vi "0036.vi"() -> ()   [LabVIEW 2014]
panel:
  out "測定中":bool
  in  "タブ制御器":enum32{"メイン画面", "設定"}(tab)
  out "XYグラフ":cluster{dbl[], dbl[]}[](graph)
  in  "再生ボタン":bool
  in  "停止ボタン":bool
  in  "全データ保存":bool
  out "経過時間":dbl format="%<%H:%M>t"
  out "数値出力":dbl format="%.1g"
  out "数値出力 2":dbl format="%.1g"
  out "数値出力 3":dbl format="%.1g"
  out "数値出力 4":dbl format="%.1g"
  out "数値出力 5":dbl format="%.1g"
  out "数値出力 6":dbl format="%.1g"
  in  "測定間隔（s）":dbl=5.0 min=5.0 step=5.0
  in  "終了時間（h）":dbl=9999.0 min=0.0 step=5.0
  out "稼働状態":bool
  out "停止合図":bool
  out "開始合図":bool
  in  "終了":bool
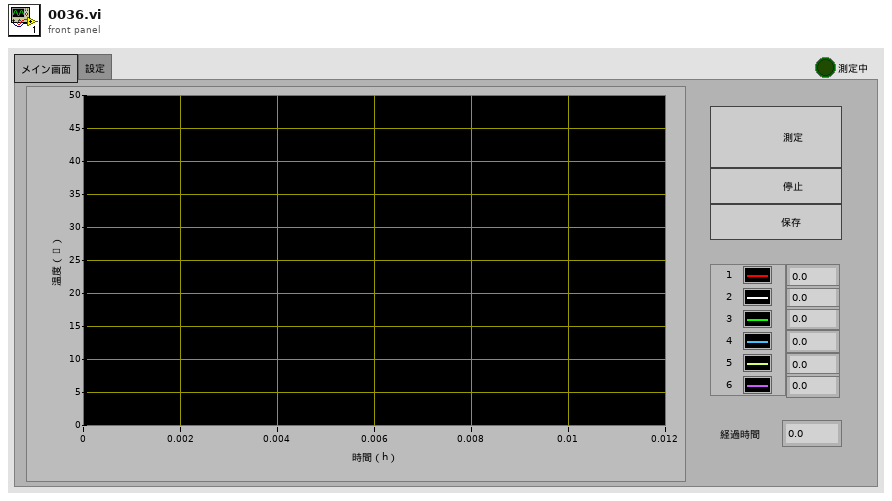
[diagram p1: front panel]
types:
  T1 = cluster{"bitRate":u32, "address":u8, "autoReadRespond":bool, "writeTimeout":u16, "readTimeout":u16, "sclLowTimeout":bool, "transferRetries":u16}
  T2 = typedef "CP2112_device.ctl" = i32
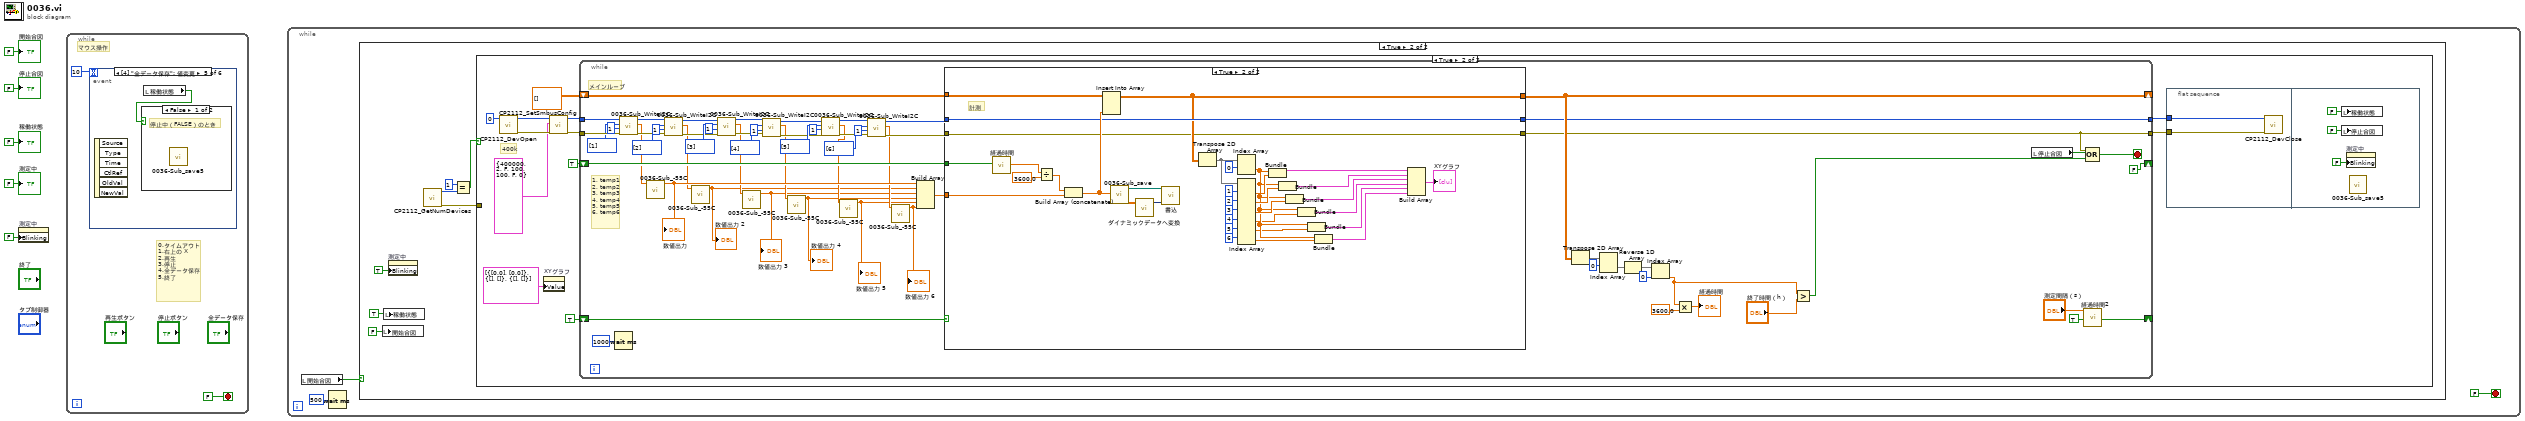
[diagram p0: block diagram]
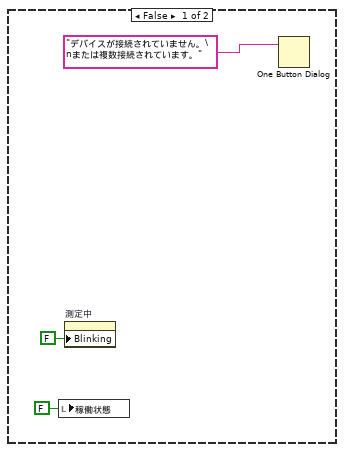
[diagram p3: hidden frame]
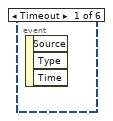
[diagram p5: hidden frame]
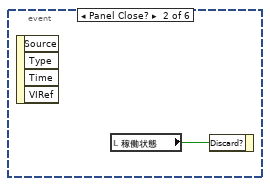
[diagram p6: hidden frame]
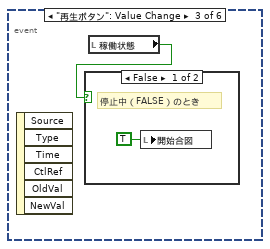
[diagram p7: hidden frame]
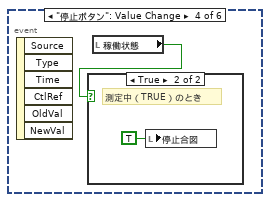
[diagram p9: hidden frame]
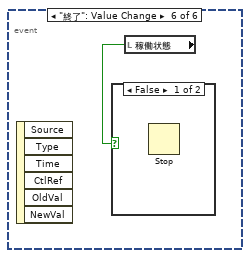
[diagram p12: hidden frame]
diagram:
  n1 = property on="測定中" class="Bool （指定）"("Blinking"=FALSE ("点滅")) -> ()  [unwired: 2 in, 2 out]
  n2 = while {
    stop <- FALSE stop-if-true
    # "マウス操作"
    # "0.タイムアウト\n1.右上の X\n2.再生\n3.停止\n4.全データ保存\n5.終了"
    n3 = event shown="[4] \"全データ保存\": 値変更" {
      selector: _ -> [_ _ _ _ _ _]
      dyn-events: _ -> [_ _ _ _ _ _]
      timeout: 10 -> [_ _ _ _ _ _]
      event Timeout {
        n4 = event-data() -> ()  [unwired: 1 in, 3 out]
      }
      event Panel Close? {
        n5 = event-data() -> ()  [unwired: 1 in, 4 out]
        n6 = local read "稼働状態"() -> (w8:bool)
        n7 = event-data("Discard?"=w8) -> ()  [unwired: 1 in, 1 out]
      }
      event "再生ボタン": Value Change {
        n8 = event-data() -> ()  [unwired: 1 in, 6 out]
        n9 = local read "稼働状態"() -> (w9:bool)
        n10 = case shown="FALSE" w9 {
          frame False {
            # "停止中（FALSE）のとき"
            n11 = local write "開始合図"(TRUE ("測定開始")) -> ()
          }
          frame True {
          }
        }
      }
      event "停止ボタン": Value Change {
        n12 = event-data() -> ()  [unwired: 1 in, 6 out]
        n13 = local read "稼働状態"() -> (w11:bool)
        n14 = case shown="TRUE" w11 {
          frame False {
          }
          frame True {
            # "測定中（TRUE）のとき"
            n15 = local write "停止合図"(TRUE ("測定開始")) -> ()
          }
        }
      }
      event "全データ保存": Value Change {
        n16 = event-data() -> ()  [unwired: 1 in, 6 out]
        n17 = local read "稼働状態"() -> (w13:bool)
        n18 = case shown="FALSE" w13 {
          frame False {
            # "停止中（FALSE）のとき"
            n19 = call "0036-Sub_save5.vi"() -> ()  [unwired: 12 in]
          }
          frame True {
          }
        }
      }
      event "終了": Value Change {
        n20 = event-data() -> ()  [unwired: 1 in, 6 out]
        n21 = local read "稼働状態"() -> (w14:bool)
        n22 = case shown="FALSE" w14 {
          frame False {
            n23 = Stop() -> ()  [unwired: 1 in]
          }
          frame True {
          }
        }
      }
    }
  }
  n24 = while {
    stop <- FALSE stop-if-true
    n25 = local read "開始合図"() -> (w16:bool)
    n26 = Wait (ms)(milliseconds to wait=u32 500 ("ミリ秒待機時間")) -> ()  [unwired: 1 out]
    n27 = case shown="TRUE" w16 {
      frame False {
      }
      frame True {
        n28 = local write "開始合図"(FALSE ("測定開始")) -> ()
        n29 = local write "稼働状態"(TRUE ("稼働状態")) -> ()
        n30 = property on="測定中" class="Bool （指定）"("Blinking"=TRUE ("点滅")) -> ()  [unwired: 2 in, 2 out]
        n31 = call <userlib>:"CP2112_GetNumDevices.vi"() -> ("error out"=w21:errorcluster, "numDevices"=w23:i32)  [unwired: 9 in, 1 out]
        n32 = Equal?(x=1, y=w23) -> (x = y?=w22:bool)
        n33 = case shown="TRUE" w22 {
          tunnel: w21 -> [_ _]
          frame False {
            n34 = local write "稼働状態"(FALSE ("稼働状態")) -> ()
            n35 = property on="測定中" class="Bool （指定）"("Blinking"=FALSE ("点滅")) -> ()  [unwired: 2 in, 2 out]
            n36 = One Button Dialog(message="デバイスが接続されていません。\nまたは複数接続されています。" ("メッセージ")) -> ()  [unwired: 1 in, 1 out]
          }
          frame True {
            # "400k"
            n37 = call <userlib>:"CP2112_DevOpen.vi"("deviceNum"=0) -> ("error out"=w35:errorcluster, "device"=w32:T2)  [unwired: 8 in, 1 out]
            n38 = property on="XYグラフ" class="XYGraph （指定）"("Value"=cluster{dbl[], dbl[]}[] [{[0.0], [0.0]}, {[], []}, {[], []}] ("XYグラフ")) -> ()  [unwired: 2 in, 2 out]
            n39 = call <userlib>:"CP2112_SetSmbusConfig.vi"("error in (no error)"=w35, "smbusInfo"=T1 {"bitRate"=400000, "address"=2, "autoReadRespond"=FALSE, "writeTimeout"=100, "readTimeout"=100, "sclLowTimeout"=FALSE, "transferRetries"=0}, "device"=w32) -> ("error out"=w34:errorcluster, "deviceOut"=w33:T2)  [unwired: 6 in, 1 out]
            n40 = while {
              tunnel: w34 -> [w95]
              tunnel: w33 -> [w96]
              tunnel: [w75] -> w39
              tunnel: [w76] -> w38
              shift-right: [w102] -> _
              shift-left: TRUE -> [w103]
              shift-right: [FALSE ("Reset")] -> _
              shift-left: TRUE ("Reset") -> [w101]
              shift-right: [w85] -> _
              shift-left: dbl[][] [] ("配列") -> [w97]
              stop <- w98 stop-if-true
              # "1, temp1\n2, temp2\n3, temp3\n4, temp4\n5, temp5\n6, temp6"
              # "メインループ"
              n41 = Wait (ms)(milliseconds to wait=u32 1000 ("ミリ秒待機時間")) -> ()  [unwired: 1 out]
              n42 = call "0036-Sub_WriteI2C.vi"("device"=w96, "書き込み"=u8[] [1], "numBytesToWrite"=u8 1, "error out"=w95) -> ("device 2"=w92:T2, "数値"=w56:dbl, "error out 2"=w93:errorcluster)  [unwired: 4 in]
              n43 = call "0036-Sub_-55C.vi"("数値入力"=w56) -> ("数値出力"=w55:dbl)  [unwired: 10 in]
              "数値出力" <- w55
              n44 = call "0036-Sub_WriteI2C.vi"("device"=w92, "書き込み"=u8[] [2], "numBytesToWrite"=u8 1, "error out"=w93) -> ("device 2"=w68:T2, "数値"=w54:dbl, "error out 2"=w67:errorcluster)  [unwired: 4 in]
              n45 = call "0036-Sub_-55C.vi"("数値入力"=w54) -> ("数値出力"=w49:dbl)  [unwired: 10 in]
              "数値出力 2" <- w49
              n46 = call "0036-Sub_WriteI2C.vi"("device"=w68, "書き込み"=u8[] [3], "numBytesToWrite"=u8 1, "error out"=w67) -> ("device 2"=w72:T2, "数値"=w53:dbl, "error out 2"=w73:errorcluster)  [unwired: 4 in]
              n47 = call "0036-Sub_-55C.vi"("数値入力"=w53) -> ("数値出力"=w48:dbl)  [unwired: 10 in]
              "数値出力 3" <- w48
              n48 = call "0036-Sub_WriteI2C.vi"("device"=w72, "書き込み"=u8[] [4], "numBytesToWrite"=u8 1, "error out"=w73) -> ("device 2"=w60:T2, "数値"=w52:dbl, "error out 2"=w59:errorcluster)  [unwired: 4 in]
              n49 = call "0036-Sub_-55C.vi"("数値入力"=w52) -> ("数値出力"=w47:dbl)  [unwired: 10 in]
              "数値出力 4" <- w47
              n50 = call "0036-Sub_WriteI2C.vi"("device"=w60, "書き込み"=u8[] [5], "numBytesToWrite"=u8 1, "error out"=w59) -> ("device 2"=w64:T2, "数値"=w51:dbl, "error out 2"=w65:errorcluster)  [unwired: 4 in]
              n51 = call "0036-Sub_-55C.vi"("数値入力"=w51) -> ("数値出力"=w46:dbl)  [unwired: 10 in]
              "数値出力 5" <- w46
              n52 = call "0036-Sub_WriteI2C.vi"("device"=w64, "書き込み"=u8[] [6], "numBytesToWrite"=u8 1, "error out"=w65) -> ("device 2"=w57:T2, "数値"=w50:dbl, "error out 2"=w58:errorcluster)  [unwired: 4 in]
              n53 = call "0036-Sub_-55C.vi"("数値入力"=w50) -> ("数値出力"=w45:dbl)  [unwired: 10 in]
              "数値出力 6" <- w45
              n54 = Build Array(w55, w49, w48, w47, w46, w45) -> (w77:dbl[])
              n55 = case shown="TRUE" w103 {
                tunnel: w58 -> [w109 w128]
                tunnel: w57 -> [w108 w133]
                tunnel: [w109 w128] -> w75
                tunnel: [w108 w133] -> w76
                tunnel: w101 -> [_ w141]
                tunnel: w97 -> [w107 w129]
                tunnel: [w107 w130] -> w85
                tunnel: w77 -> [_ w126]
                frame False {
                }
                frame True {
                  # "計測"
                  n56 = call "経過時間"("Reset"=w141) -> ("Elapsed Time (s)"=w139:dbl)  [unwired: 11 in, 7 out]
                  n57 = Divide(x=w139, y=3600.0) -> (x/y=w138:dbl)
                  n58 = Build Array (concatenate)(w138, w126) -> (w137:dbl[])
                  n59 = Insert Into Array(array=w129, new element=w137) -> (w130:dbl[][])  [unwired: 2 in]
                  n60 = call "0036-Sub_save.vi"("部分配列 2"=w137) -> ("パス"=w144:path, "転置配列"=w142:dbl[][])  [unwired: 8 in]
                  n61 = call "ダイナミックデータへ変換"("2D Array"=w142) -> ("Dynamic Data Type"=w143:dynamicdata)  [unwired: 3 in]
                  n62 = call "書込"("Signals"=w143, "Filename"=w144) -> ()  [unwired: 15 in, 3 out]
                  n63 = Transpose 2D Array(2D array=w130) -> (transposed array=w127:dbl[][])
                  n64 = Index Array(array=w127, index (row)=0 ("指標 （行）")) -> (element=w118:dbl[])  [unwired: 1 in]
                  n65 = Index Array(array=w127, index (row) #1=1 ("指標 （行）"), index (row) #2=2 ("指標 （行）"), index (row) #3=3 ("指標 （行）"), index (row) #4=4 ("指標 （行）"), index (row) #5=5 ("指標 （行）"), index (row) #6=6 ("指標 （行）")) -> (element #1=w134:dbl[], element #2=w120:dbl[], element #3=w119:dbl[], element #4=w117:dbl[], element #5=w116:dbl[], element #6=w115:dbl[])  [unwired: 6 in]
                  n66 = Bundle(w118, w134) -> (w132:cluster{dbl[], dbl[]})  [unwired: 1 in]
                  n67 = Bundle(w118, w120) -> (w114:cluster{dbl[], dbl[]})  [unwired: 1 in]
                  n68 = Bundle(w118, w119) -> (w113:cluster{dbl[], dbl[]})  [unwired: 1 in]
                  n69 = Bundle(w118, w117) -> (w112:cluster{dbl[], dbl[]})  [unwired: 1 in]
                  n70 = Bundle(w118, w116) -> (w111:cluster{dbl[], dbl[]})  [unwired: 1 in]
                  n71 = Bundle(w118, w115) -> (w110:cluster{dbl[], dbl[]})  [unwired: 1 in]
                  n72 = Build Array(w132, w114, w113, w112, w111, w110) -> (→"XYグラフ":cluster{dbl[], dbl[]}[])
                }
              }
              n73 = Transpose 2D Array(2D array=w85) -> (transposed array=w90:dbl[][])
              n74 = Index Array(array=w90, index (row)=0 ("指標 （行）")) -> (element=w87:dbl[])  [unwired: 1 in]
              n75 = Reverse 1D Array(array=w87) -> (reversed array=w86:dbl[])
              n76 = Index Array(array=w86, index=0 ("指標")) -> (element=w79:dbl)
              n77 = Multiply(x=w79, y=3600.0) -> (x*y=→"経過時間":dbl)
              n78 = Greater?(x=w79, y="終了時間（h）") -> (0:w78:bool)
              n79 = local read "停止合図"() -> (w99:bool)
              n80 = call "経過時間2"("Time Target (s)"="測定間隔（s）", "Auto Reset"=TRUE) -> ("Time has Elapsed"=w102:bool)  [unwired: 10 in, 7 out]
              n81 = Compound Arithmetic op=OR(w75, w99, w78) -> (w98:bool)
            }
            n82 = flat-sequence {
              tunnel: w39 -> [w41]
              tunnel: w38 -> [w40]
              frame #0 {
                n83 = call <userlib>:"CP2112_DevClose.vi"("error in (no error)"=w41, "device"=w40) -> ()  [unwired: 9 in, 1 out]
              }
              frame #1 {
                n84 = local write "稼働状態"(FALSE ("稼働状態")) -> ()
                n85 = local write "停止合図"(FALSE ("停止合図")) -> ()
                n86 = property on="測定中" class="Bool （指定）"("Blinking"=FALSE ("点滅")) -> ()  [unwired: 2 in, 2 out]
                n87 = call "0036-Sub_save5.vi"() -> ()  [unwired: 12 in]
              }
            }
          }
        }
      }
    }
  }
  "開始合図" <- FALSE ("測定開始")
  "停止合図" <- FALSE ("測定停止")
  "稼働状態" <- FALSE ("稼働状態")
  "測定中" <- FALSE ("測定中")
